vi "Emit.vi"(8 "error in (no error)":errorcluster, 10 "response":T1, 11 "BaseResponder in":refnum<class "BaseResponder.lvclass">) -> (0 "error out":errorcluster, 3 "BaseResponder out":refnum<class "BaseResponder.lvclass">)   [LabVIEW 2013, in "BaseResponder.lvclass"]
doc: "Emit a response to the owning application"
uses:
  BaseResponder.lvclass
  response.ctl
  driver_status.ctl
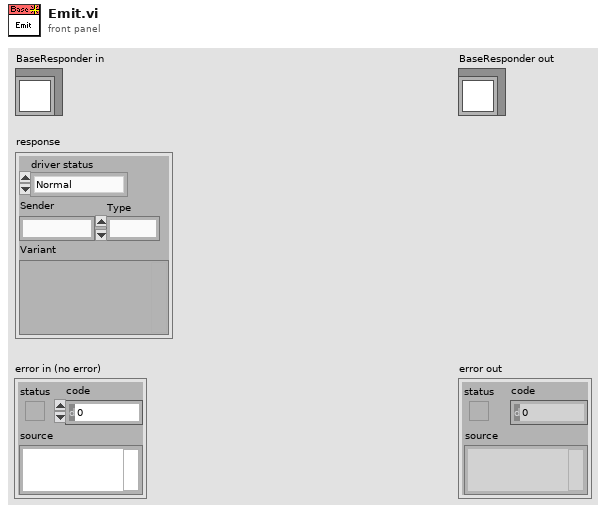
[diagram p1: front panel]
types:
  T1 = typedef "response.ctl" = cluster{"driver status":T2, "Sender":string, "Type":i32, "Variant":variant}
  T2 = typedef "driver_status.ctl" = enum16{"Normal", "Startup", "Connection lost", "Reconnected", "Timeout", "Idle", "Busy"}
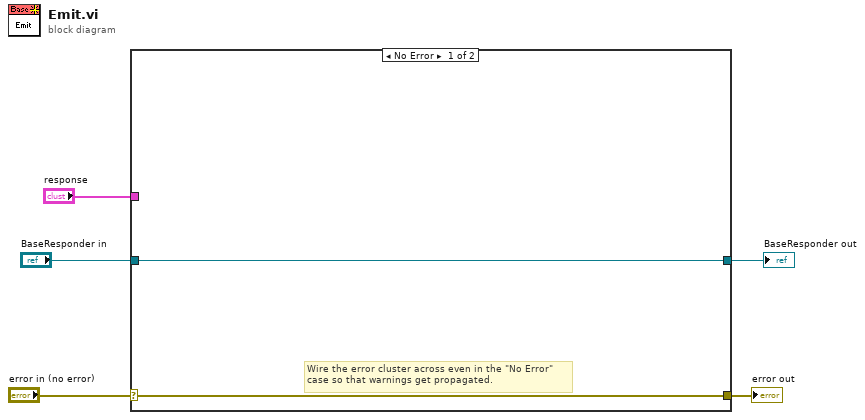
[diagram p0: block diagram]
diagram:
  n1 = case shown="No Error" "error in (no error)" {
    selector: "error in (no error)" -> [w7 w9]
    tunnel: [w7 w9] -> w4
    tunnel: [w6 w8] -> w2
    tunnel: "BaseResponder in" -> [w6 w8]
    tunnel: "response" -> [_ _]
    frame No Error {
      # "Wire the error cluster across even in the \"No Error\"\ncase so that warnings get propagated."
    }
    frame Error {
    }
  }
  "error out" <- w4
  "BaseResponder out" <- w2
